vi "Prepare Results.vi"(8 "error in (no error)":errorcluster, 9 "Execution Time":dbl, 11 "LUnit Test Case In":refnum<class "LUnit Test Case.lvclass">) -> (0 "error out":errorcluster, 2 "Results":T1[](array[typedef]), 3 "LUnit Test Case Out":refnum<class "LUnit Test Case.lvclass">)   [LabVIEW 2020, in "LUnit Test Case.lvclass"]
uses:
  LUnit Test Case.lvclass
  Result/Type.ctl
  Result/Result.lvlib
  Result/Status.ctl
  Result/Result.ctl
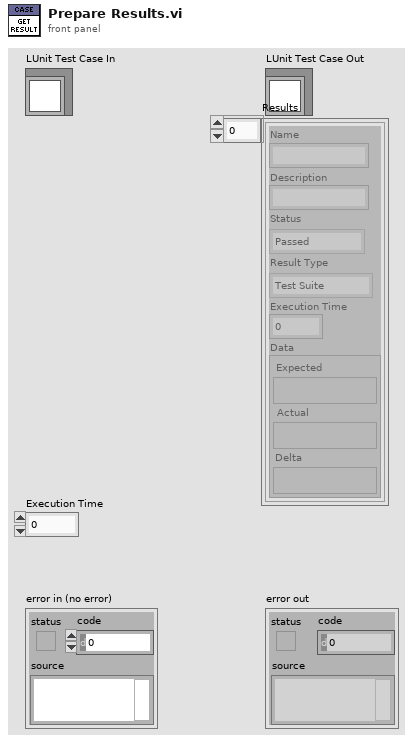
[diagram p1: front panel]
types:
  T1 = typedef "Result.lvlib/Result.ctl" = cluster{"Name":string, "Description":string, "Status":T2, "Result Type":T3, "Execution Time":dbl, "Data":cluster{"Expected":variant, "Actual":variant, "Delta":variant}}
  T2 = typedef "Result.lvlib/Status.ctl" = enum16{"", "Passed", "Failed", "Error", "Skipped", "Setup Error", "Broken", "Teardown Error"}
  T3 = typedef "Result.lvlib/Type.ctl" = enum16{"Test Case", "Test Suite", "Test Run", "Pass", "Fail", "Skip", "Pass if", "Fail if", "Pass if Error", "Fail if Error", "Pass if Equal", "Fail if Equal"}
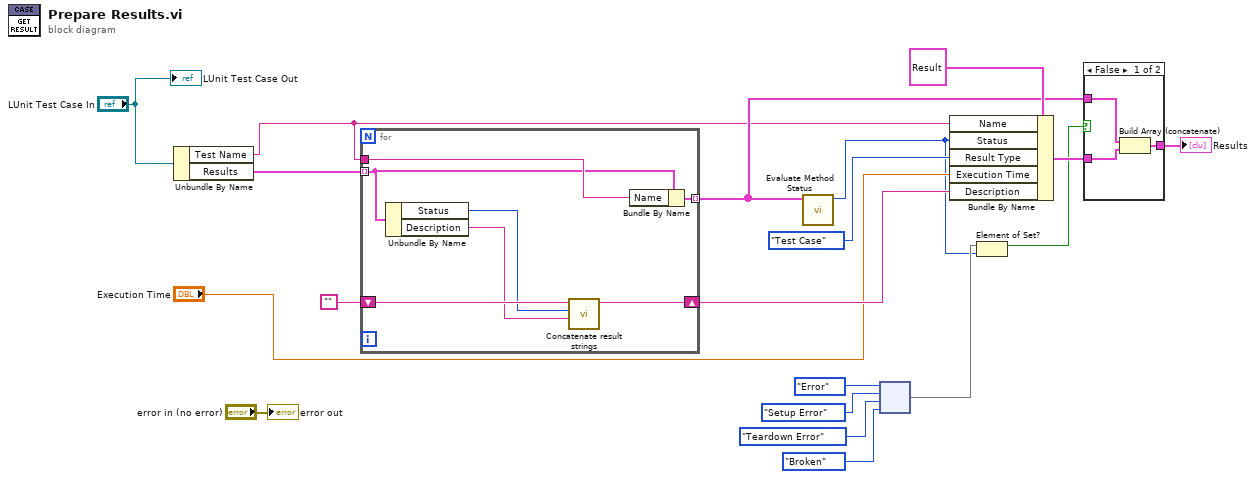
[diagram p0: block diagram]
diagram:
  n1 = Unbundle By Name("LUnit Test Case In") -> ("Test Name"=w1:string, "Results"=w18:T1[])
  n2 = for {
    tunnel: w18 -> [w23] mode=indexing
    tunnel: w1 -> [w26]
    tunnel: [w25] -> w15 mode=indexing
    shift-right: [w20] -> w10
    shift-left: "" ("Input String") -> [w24]
    n3 = Unbundle By Name(w23) -> ("Status"=w22:T2, "Description"=w21:string)
    n4 = call "Concatenate result strings.vi"("Description"=w21, "Status"=w22, "Input String"=w24) -> ("Output String"=w20:string)  [unwired: 8 in]
    n5 = Bundle By Name(cluster=w23, "Name"=w26) -> (w25:T1)
  }
  n6 = call "Evaluate Method Status.vi"("Results"=w15) -> ("Status"=w3:T2)  [unwired: 10 in]
  n7 = node(Status."Error" ("Status"), Status."Setup Error" ("Status"), Status."Teardown Error" ("Status"), Status."Broken" ("Status")) -> (w4:set{T2})
  n8 = Bundle By Name(cluster=T1 {"Name"="", "Description"="", "Status"=enum."Passed", "Result Type"=enum."Test Case", "Execution Time"=0.0, "Data"={"Expected"=variant, "Actual"=variant, "Delta"=variant}} ("Results"), "Name"=w1, "Status"=w3, "Result Type"=Type."Test Case", "Execution Time"="Execution Time", "Description"=w10) -> (w13:T1)
  n9 = Element of Set?(10:w3, 11:w4) -> (3:w2:bool)
  n10 = case shown="False" w2 {
    tunnel: w15 -> [w29 w30]
    tunnel: [w28 w30] -> w14
    tunnel: w13 -> [w27 _]
    frame False {
      n11 = Build Array (concatenate)(w29, w27) -> (w28:T1[])
    }
    frame True {
    }
  }
  "Results" <- w14
  "error out" <- "error in (no error)"
  "LUnit Test Case Out" <- "LUnit Test Case In"
